vi "Save data.vi"(8 "error in (no error)":errorcluster, 10 "Data":T3, 11 "file refs":T1 {"file" format="%.0x"}) -> (0 "error out":errorcluster, 3 "file refs out":T1 {"file" format="%.0x"})   [LabVIEW 2012]
uses:
  File refs.ctl
  <vilib>/addons/h5labview2/base/hid_t.ctl
  Data.ctl
  Treatment.ctl
  Treatment type.ctl
  HDF5 append data (DBL 2D).vi
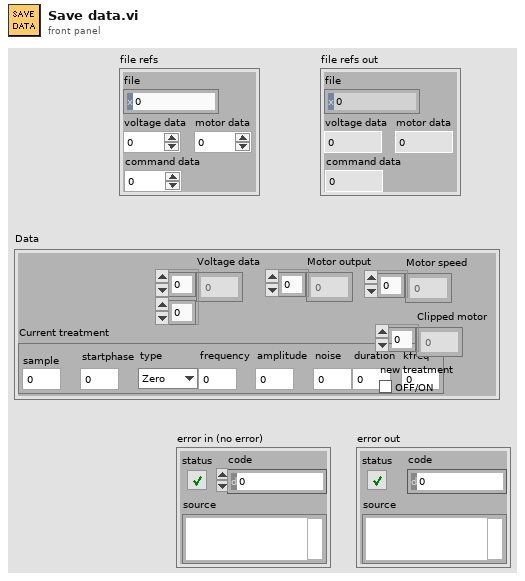
[diagram p1: front panel]
types:
  T1 = typedef "File refs.ctl" = cluster{"file":T2, "voltage data":i32, "motor data":i32, "command data":i32}
  T2 = typedef "hid_t.ctl" = i32
  T3 = typedef "Data.ctl" = cluster{"Voltage data":dbl[][], "Motor output":dbl[], "Current treatment":T4, "Motor speed":dbl[], "Clipped motor":dbl[], "new treatment":bool}
  T4 = typedef "Treatment.ctl" = cluster{"sample":dbl, "startphase":dbl, "type":T5, "frequency":dbl, "amplitude":dbl, "noise":dbl, "duration":dbl, "kfreq":dbl}
  T5 = typedef "Treatment type.ctl" = enum16{"Zero", "Sine", "Frequency sweep"}
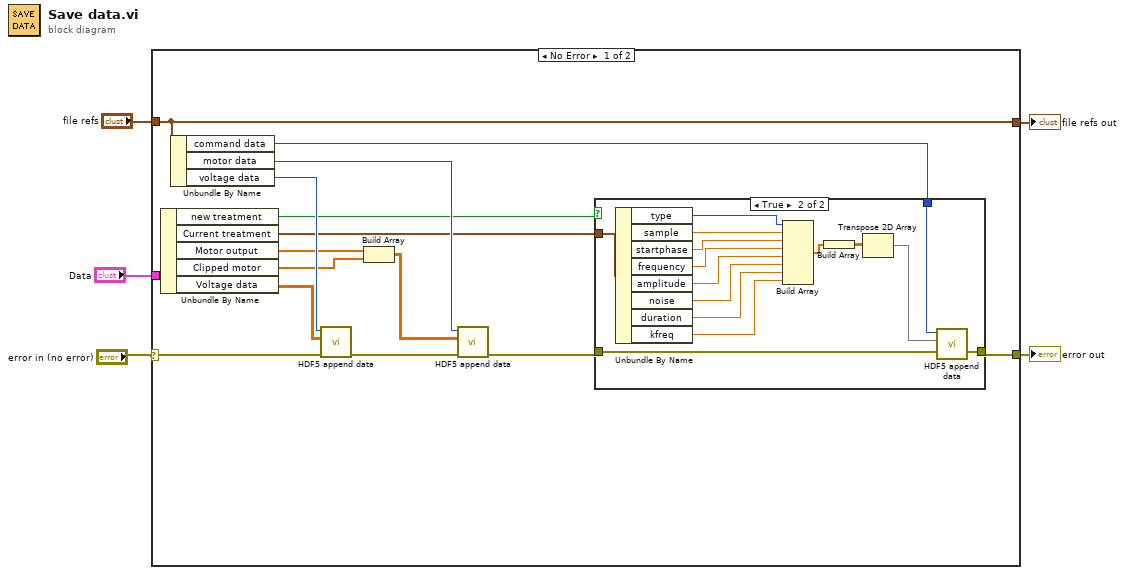
[diagram p0: block diagram]
diagram:
  n1 = case shown="No Error" "error in (no error)" {
    selector: "error in (no error)" -> [w19 w37]
    tunnel: "file refs" -> [w13 w38]
    tunnel: "Data" -> [w18 _]
    tunnel: [w8 w37] -> w2
    tunnel: [w13 w38] -> w1
    frame No Error {
      n2 = Unbundle By Name(w18) -> ("new treatment"=w6:bool, "Current treatment"=w11:T4, "Motor output"=w15:dbl[], "Clipped motor"=w7:dbl[], "Voltage data"=w17:dbl[][])
      n3 = Unbundle By Name(w13) -> ("command data"=w10:i32, "motor data"=w14:i32, "voltage data"=w20:i32)
      n4 = call-poly "HDF5 append data.vi"("error in (no error)"=w19, "data"=w17, "dset in"=w20) -> ("error out"=w16:errorcluster)  [unwired: 7 in, 1 out]
      n5 = Build Array(w15, w7) -> (w12:dbl[][])
      n6 = call-poly "HDF5 append data.vi"("error in (no error)"=w16, "data"=w12, "dset in"=w14) -> ("error out"=w9:errorcluster)  [unwired: 7 in, 1 out]
      n7 = case shown="True" w6 {
        tunnel: w11 -> [_ w36]
        tunnel: w10 -> [_ w28]
        tunnel: w9 -> [w21 w27]
        tunnel: [w21 w26] -> w8
        frame False {
        }
        frame True {
          n8 = Unbundle By Name(w36) -> ("type"=w22:T5, "sample"=w35:dbl, "startphase"=w34:dbl, "frequency"=w33:dbl, "amplitude"=w32:dbl, "noise"=w25:dbl, "duration"=w24:dbl, "kfreq"=w23:dbl)
          n9 = Build Array(w22, w35, w34, w33, w32, w25, w24, w23) -> (w31:dbl[])
          n10 = Build Array(w31) -> (w30:dbl[][])
          n11 = Transpose 2D Array(2D array=w30) -> (transposed array=w29:dbl[][])
          n12 = call-poly "HDF5 append data.vi"("error in (no error)"=w27, "data"=w29, "dset in"=w28) -> ("error out"=w26:errorcluster)  [unwired: 7 in, 1 out]
        }
      }
    }
    frame Error {
    }
  }
  "error out" <- w2
  "file refs out" <- w1
